vi "monitor error id str.vi"(11 "error_id":u32(ring) items=["E_OK", "E_EVENT_OVERFLOW", "E_BUFFER_OVERFLOW", "E_SD_RESPONSE_TIMEOUT", "E_SD_R1_INVALID", "E_SD_R1_PARAM_ERROR", "E_SD_R1_ADDRESS_ERROR", "E_SD_R1_ERASE_SEQ_ERROR", "E_SD_R1_CRC_ERROR", "E_SD_R1_ILLEGAL_CMD", "E_SD_R1_ERASE_RESET", "E_SD_CMD_0", "E_SD_CMD_8", "E_SD_CMD_55", "E_SD_CMD_41", "E_SD_CMD_16", "E_SD_CMD_24", "E_SD_CMD_17", "E_SD_CMD_9", "E_SD_CMD_OTHER", "E_SD_BAD_SIZE", "E_SD_STATE", "E_SD_BUFFER_FULL", "E_SD_CMD_8_FORMAT", "E_SD_CMD_8_VOLTAGE", "E_SD_CMD_8_CHECK", "E_SD_WRITE_CRC", "E_SD_READ_CRC", "E_SD_CSD_CRC", "E_SD_WRITE_ERROR", "E_SD_WRITE_OTHER", "E_SD_PROCESS", "E_UART_COLLISION", "E_DECIMATE_OVERFLOW1", "E_DECIMATE_OVERFLOW2", "E_DECIMATE_NEG1", "E_DECIMATE_NEG2", "E_WIRELESS_BUFFER_OVERFLOW", "E_SPI_TIMEOUT", "E_DEBUG_1", "E_DEBUG_2", "E_DEBUG_3", "E_DEBUG_4", "E_DEBUG_5", "E_DEBUG_6", "E_DEBUG_7", "E_DEBUG_8", "E_DEBUG_9", "E_DEBUG_10", "E_DEBUG_11", "E_DEBUG_12", "E_DEBUG_13", "E_DEBUG_14", "E_DEBUG_15", "E_DEBUG_16", "E_OSC_FAULT", "E_DCO_FAULT", "E_LF_FAULT", "E_XT1_FAULT", "E_OFF_BATTERY", "E_OFF_SPIN", "E_OFF_ALWAYS", "E_OFF_WIRELESS", "E_OFF_HALT", "E_WDT_RESET", "E_INVALID_CONFIG", "E_DEBUG_17", "E_DEBUG_18", "E_DEBUG_19", "E_DEBUG_20", "E_DEBUG_21", "E_DEBUG_22", "E_DEBUG_23", "E_DEBUG_24", "E_DEBUG_25", "E_DEBUG_26", "E_DEBUG_27", "E_DEBUG_28", "E_DEBUG_29", "E_DEBUG_30", "E_DEBUG_31", "E_DEBUG_32", "E_ISR_OVER_RUN", "E_STANDBY"]) -> (3 "function return":string)   [LabVIEW 2019, in "apdm.lvlib"]
doc: "APDM_EXPORT const char* apdm_monitor_error_id_str(const apdm_monitor_error_id_t error_id);"
uses:
  apdm.lvlib
  Lee Lab/CP FES Walking 2018/Code/Working/LabVIEW/apdm.dll
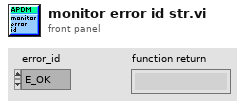
[diagram p1: front panel]
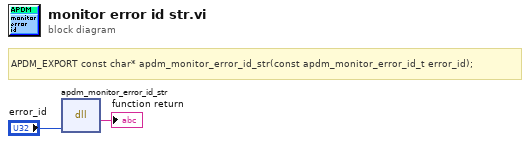
[diagram p0: block diagram]
diagram:
  # "APDM_EXPORT const char* apdm_monitor_error_id_str(const apdm_monitor_error_id_t error_id);"
  n1 = dll-call lib="C:/Users/jfalesi/Dropbox/Lee Lab/CP FES Walking 2018/Code/Working/LabVIEW/apdm.*" fn="apdm_monitor_error_id_str"("error_id"="error_id") -> (→"function return":string)  [unwired: 4 in, 2 out]
